vi "Calibration Parameter Filter.vi"(7 "Parameter_List":string[](array[string]), 11 "XML Data In":T1[](array[typedef])) -> (3 "XML Data Out":T1[](array[typedef]))   [LabVIEW 2010]
uses:
  Calibration dates.ctl
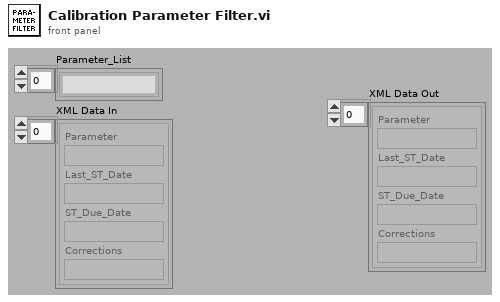
[diagram p1: front panel]
types:
  T1 = typedef "Calibration dates.ctl" = cluster{"Parameter":string, "Last_ST_Date":string, "ST_Due_Date":string, "Corrections":string}
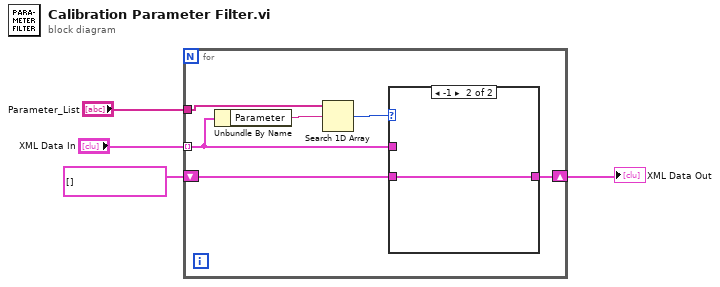
[diagram p0: block diagram]
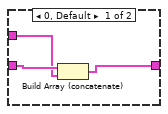
[diagram p2: hidden frame]
diagram:
  n1 = for {
    tunnel: "XML Data In" -> [w6] mode=indexing
    shift-right: [w5] -> w1
    shift-left: T1[] [] ("XML File Data") -> [w7]
    tunnel: "Parameter_List" -> [w10]
    n2 = Unbundle By Name(w6) -> ("Parameter"=w9:string)
    n3 = Search 1D Array(1D array=w10, element=w9) -> (index of element=w8:i32)  [unwired: 1 in]
    n4 = case shown="-1" w8 {
      tunnel: w7 -> [w13 w14]
      tunnel: w6 -> [w12 _]
      tunnel: [w11 w14] -> w5
      frame 0, Default {
        n5 = Build Array (concatenate)(w13, w12) -> (w11:T1[])
      }
      frame -1 {
      }
    }
  }
  "XML Data Out" <- w1
